vi "Copy Linked List Attributes.vi"(7 "Sink Linked List ID":string, 8 "error in (no error)":errorcluster, 10 "Source Linked List ID":string, 11 "Linked List Ref":refnum<data-value>) -> (0 "error out":errorcluster, 3 "Linked List Ref out":refnum<data-value>)   [LabVIEW 2019, in "Linked Lists.lvlib" / "Linked List Ref.lvclass"]
uses:
  <vilib>/gpm_packages/@cs/linked-list/Source/Linked List/Linked List Ref/Linked List Ref.lvclass
  <vilib>/gpm_packages/@cs/linked-list/Source/Linked List/ILinkedList/ILinked List.lvclass
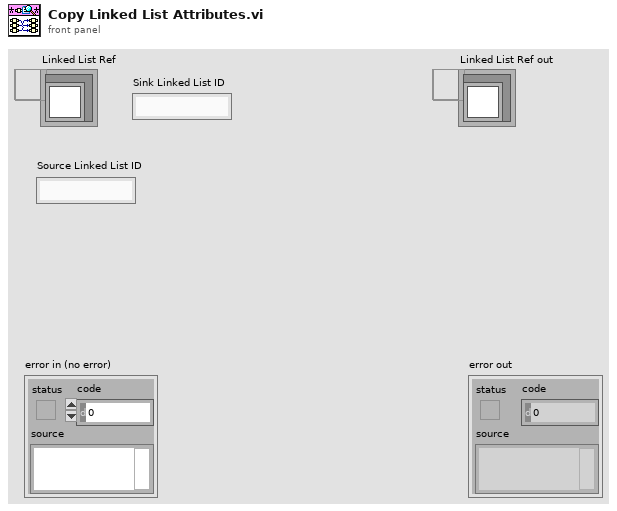
[diagram p1: front panel]
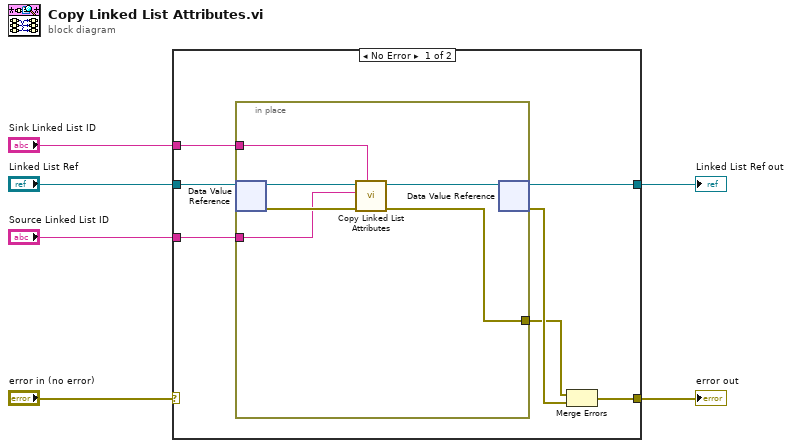
[diagram p0: block diagram]
diagram:
  n1 = case shown="No Error" "error in (no error)" {
    selector: "error in (no error)" -> [_ w21]
    tunnel: "Linked List Ref" -> [w13 w20]
    tunnel: "Sink Linked List ID" -> [w12 _]
    tunnel: "Source Linked List ID" -> [w11 _]
    tunnel: [w9 w21] -> w2
    tunnel: [w10 w20] -> w1
    frame No Error {
      n2 = in-place {
        in-place-border: w12 -> [w18]
        in-place-border: w11 -> [w14]
        in-place-border: [w15] -> w7
        n3 = in-place-dvr #1(w13) -> (w19:refnum<class "ILinked List.lvclass">, w16:errorcluster)
        n4 = call-dynamic "Copy Linked List Attributes.vi"("Sink Linked List ID"=w18, "error in (no error)"=w16, "Source Linked List ID"=w14, "ILinked List in"=w19) -> ("error out"=w15:errorcluster, "ILinked List out"=w17:refnum<class "ILinked List.lvclass">)  [unwired: 6 in]
        n5 = in-place-dvr #1(w17) -> (w10:refnum<data-value>, w8:errorcluster)
      }
      n6 = Merge Errors(w7, w8) -> (w9:errorcluster)
    }
    frame Error {
    }
  }
  "error out" <- w2
  "Linked List Ref out" <- w1
